vi "Wait Scan_Rf.vi"(8 "error in (no error)":errorcluster, 10 "OK&NG":refnum<vi>, 11 "Data In":T2) -> (0 "error out":errorcluster, 1 "States":T1, 3 "Data Out":T2)   [LabVIEW 2014]
doc: "Use this template to build a standard state machine design pattern. Each state executes code and determines which state to transition to. Contrast this design pattern with the User Interface Event Handler pattern, in which code executes in response to user actions. Contrast this design pattern also with the Queued Message Handler pattern, in which each message handling code can queue zero or more new messages.\nNote: This template does not contain the most recent programming guidelines recommended by National Instruments. For a complete, project-based implementation of the Standard State Machine pattern, use the Create Project dialog box instead of this template."
uses:
  controls/Wait Scan States.ctl
  controls/Data.ctl
  controls/State.ctl
panel:
  # "日期"
  # "機種名稱"
  # "機種代號"
  # "商品條碼"
  # "台"
  # "OK"
  # "NG"
  # "台"
  # "總計"
  # "台"
  # "日期"
  # "機種名稱"
  # "機種代號"
  # "商品條碼"
  # "台"
  # "OK"
  # "NG"
  # "台"
  # "總計"
  # "台"
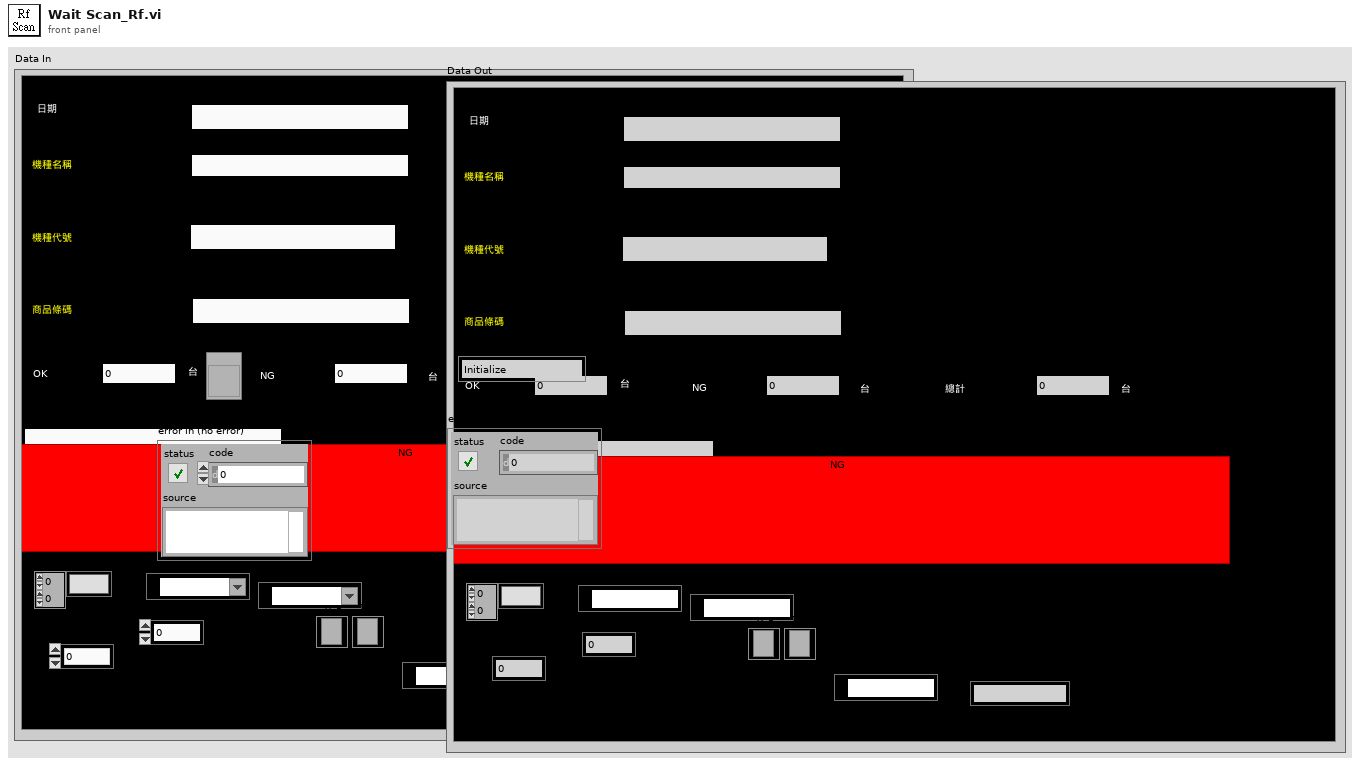
[diagram p1: front panel]
types:
  T1 = typedef "State.ctl" = enum16{"Initialize", "Wait for Scan", "State 1", "State 2", "NG", "NG1", "OK", "OKNG", "OKNG1", "Exit"}
  T2 = typedef "Data.ctl" = cluster{"Date":string, "BarCode1":string, "BarCode2":string, "BarCode3":string, "Message":string, "OK Count":u16, "NG Count":u16, "Total Count":u16, "ModelData":string[][], "OK&NG":bool, "COM1":refnum<visa-resource-name>, "COM2":refnum<visa-resource-name>, "IO":i32, "Time":u32, "TCP":refnum<k5>, "TCP 2":refnum<k5>, "COM3":refnum<visa-resource-name>, "CheckPars":string}
  T3 = typedef "Wait Scan States.ctl" = enum16{"Initialize", "State1", "Stop"}
  T4 = typedef "Data1.ctl" = cluster{"Date":string, "BarCode1":string, "BarCode2":string, "BarCode3":string, "Message":string, "OK Count":u16, "NG Count":u16, "Total Count":u16, "ModelData":string[][], "OK&NG":bool, "COM1":refnum<visa-resource-name>, "COM2":refnum<visa-resource-name>, "IO":i32, "Time":u32, "TCP":refnum<k5>, "TCP 2":refnum<k5>, "COM1 2":refnum<visa-resource-name>, "CheckNum":string, "BarCode1_1":string, "BarCode2_1":string, "BarCode3_1":string, "日期":string, "機種":string, "機號":string, "商品條碼1":string, "OK_1":string, "OK":string, "NG":string, "NG_1":string, "Total":string, "Total_1":string, "ClaerTime":u32, "Pjson":T5, "LotNo":string[], "CheckParsArray":string[], "BarCode4":string, "BarCode4_1":string, "商品條碼2":string, "BarCode5":string, "BarCode5_1":string, "商品條碼3":string, "ReScanNG":i32, "NGTimeCT":u32}
  T5 = typedef "Payjson.ctl" = cluster{"DEPT":string, "LINE":string, "STANO":string, "WORKNO":string, "PRODSN":string, "COMPNTID":string, "COMPNTLOT":string, "COMPNTSN":string, "USEDQTY":i16, "OPDATE":string, "OPUSER":string, "RECVDATE":string, "MMODU":string}[]
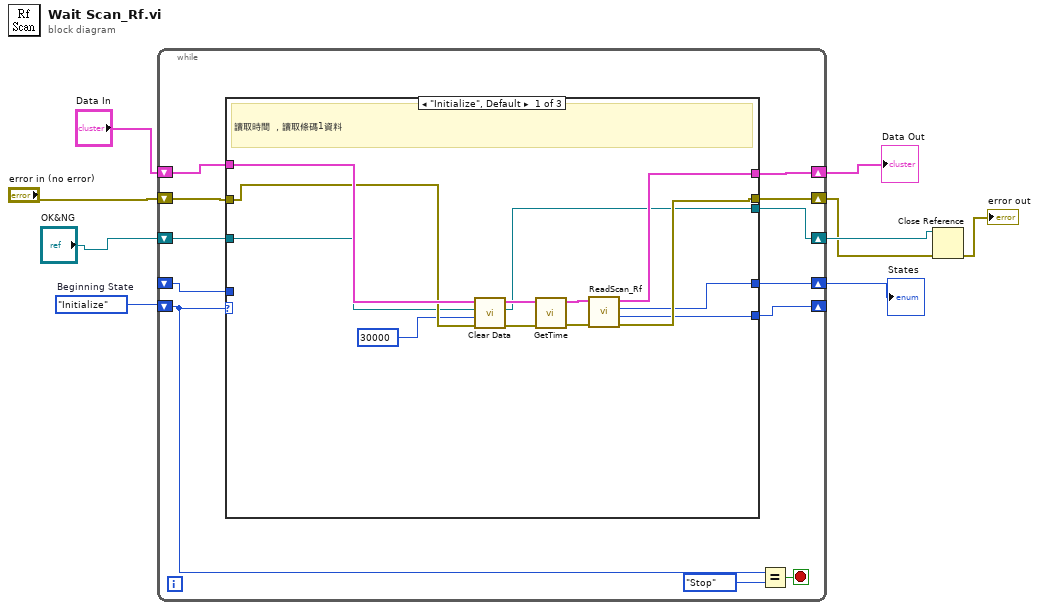
[diagram p0: block diagram]
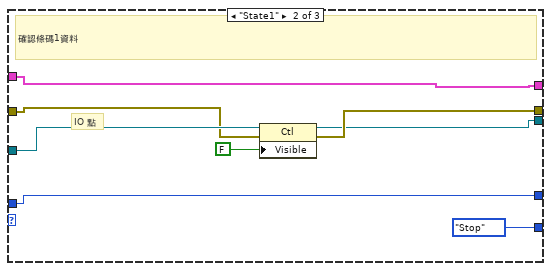
[diagram p2: hidden frame]
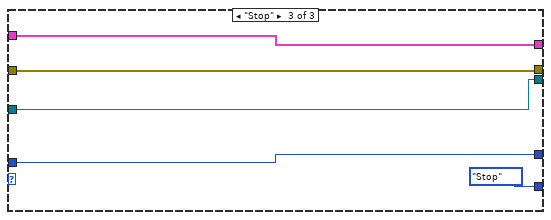
[diagram p3: hidden frame]
diagram:
  w9 = Wait_Scan_States."Initialize"  # Beginning State
  n1 = while {
    shift-right: [w18] -> _
    shift-left: w9 -> [w19]
    shift-right: [w15] -> w7
    shift-left: "Data In" -> [w17]
    shift-right: [w14] -> w3
    shift-left: "error in (no error)" -> [w16]
    shift-right: [w13] -> w5
    shift-left: _ -> [w12]
    shift-right: [w10] -> w4
    shift-left: "OK&NG" -> [w11]
    stop <- w21 stop-if-true
    n2 = case shown="\"Initialize\", Default" w19 {
      tunnel: [w29 Wait_Scan_States."Stop" ("Next State") Wait_Scan_States."Stop" ("Next State")] -> w18
      tunnel: w17 -> [w28 w35 w44]
      tunnel: w16 -> [w26 w34 w43]
      tunnel: [w31 w35 w44] -> w15
      tunnel: [w32 w38 w43] -> w14
      tunnel: [w30 w36 w45] -> w13
      tunnel: w12 -> [_ w36 w45]
      tunnel: w11 -> [w22 w39 w42]
      tunnel: [w24 w37 w42] -> w10
      frame "Initialize", Default {
        # "讀取時間 ，讀取條碼1資料"
        n3 = call "Clear Data.vi"("Data In"=w28, "Clust Refnum"=w22, "Time"=u32 30000, "error in (no error)"=w26) -> ("Data Out"=w27:T4, "Clust Refnum"=w24:refnum<vi>, "error out"=w25:errorcluster)  [unwired: 4 in]
        n4 = call "GetTime.vi"("Data In"=w27) -> ("Data Out"=w33:T4)  [unwired: 10 in]
        n5 = call "ReadScan_Rf.vi"("error in (no error)"=w25, "Data In"=w33) -> ("error out"=w32:errorcluster, "Next State"=w29:T3, "States"=w30:T1, "Data Out"=w31:T2)  [unwired: 6 in]
      }
      frame "State1" {
        # "IO 點"
        # "確認條碼1資料"
        n6 = property class="Ctl"(reference=w39, error in=w34, "Visible"=FALSE) -> (reference out=w37:refnum<vi>, error out=w38:errorcluster)
      }
      frame "Stop" {
      }
    }
    n7 = Equal?(x=w19, y=Wait_Scan_States."Stop" ("States")) -> (x = y?=w21:bool)
  }
  "Data Out" <- w7
  "States" <- w5
  n8 = Close Reference(reference=w4, error in (no error)=w3) -> (error out=→"error out":errorcluster)
